vi "setTiming.vi"(8 "error in (no error)":errorcluster, 11 "niDAQmxDO in":refnum<class "niDAQmxDO.lvclass">) -> (0 "error out":errorcluster, 3 "niDAQmxDO out":refnum<class "niDAQmxDO.lvclass">)   [LabVIEW 2009, in "Hardware.lvlib" / "Channels.lvlib" / "niDAQmxDO.lvclass"]
doc: "need to add routings."
uses:
  niDAQmxDO.lvclass
  <vilib>/DAQmx/configure/timing.llb/DAQmx Timing (Sample Clock).vi
  C:/Program Files/National Instruments/LabVIEW 2009/resource/objmgr/daqmx.rc
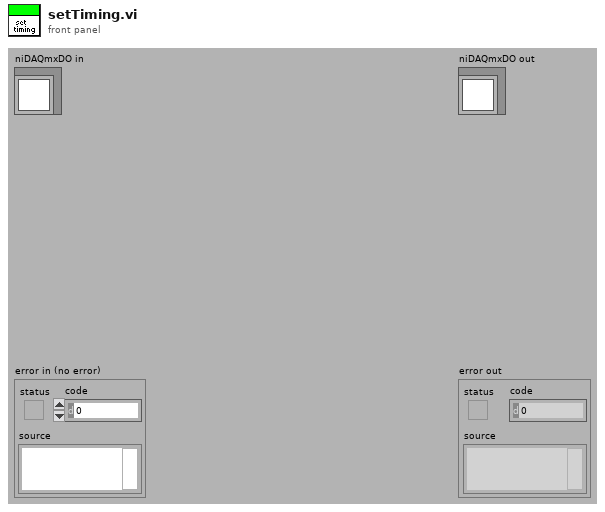
[diagram p1: front panel]
types:
  T1 = cluster{"Master Clock source":string, "Master Clock rate":dbl, "Start trigger line":string, "Scan rate":dbl, "Stop trigger line":string, "Sample Number":dbl}
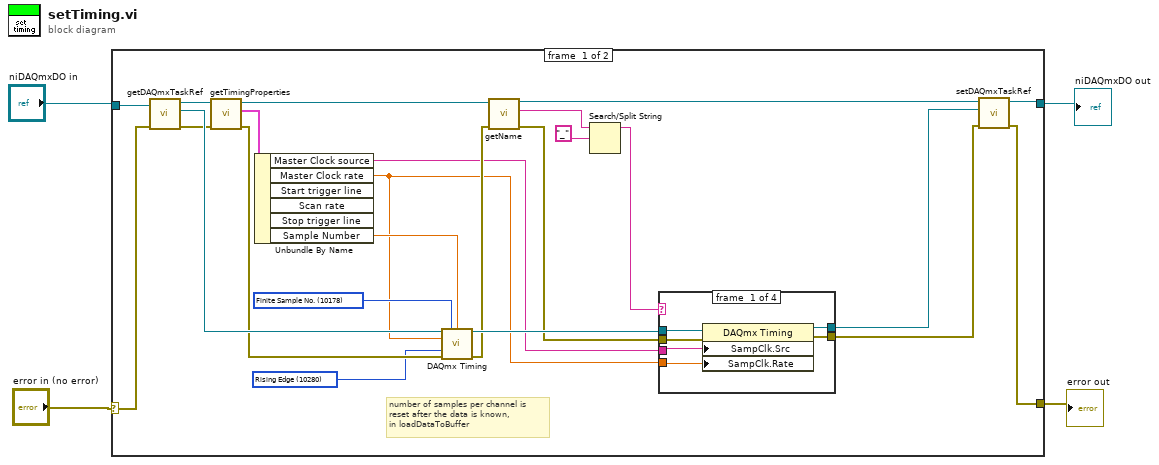
[diagram p0: block diagram]
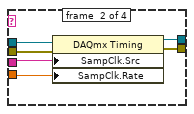
[diagram p2: hidden frame]
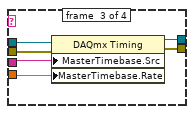
[diagram p3: hidden frame]
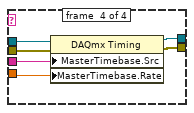
[diagram p4: hidden frame]
diagram:
  n1 = case shown="No Error" "error in (no error)" {
    selector: "error in (no error)" -> [w27 w54]
    tunnel: "niDAQmxDO in" -> [w28 w53]
    tunnel: [w20 w54] -> w2
    tunnel: [w19 w53] -> w1
    frame #0 {
      w16 = u16 10280 items=["Rising Edge"=10280]
      w22 = u16 10178 items=["Finite Sample No."=10178]
      # "number of samples per channel is\nreset after the data is known,\nin loadDataToBuffer"
      n2 = call "getDAQmxTaskRef.vi"("error in (no error)"=w27, "niDAQmxDO.lvclass in"=w28) -> ("error out"=w24:errorcluster, "DAQmx Task Ref"=w26:refnum<k21>, "niDAQmxDO.lvclass out"=w25:refnum<class "niDAQmxDO.lvclass">)  [unwired: 7 in]
      n3 = call-dynamic "getTimingProperties.vi"("error in (no error)"=w24, "DigitalOutput.lvclass in"=w25) -> ("error out"=w21:errorcluster, "Timing"=w23:T1, "DigitalOutput.lvclass out"=w15:refnum<class "niDAQmxDO.lvclass">)  [unwired: 7 in]
      n4 = Unbundle By Name(w23) -> ("Master Clock source"=w7:string, "Master Clock rate"=w11:dbl, "Sample Number"=w18:dbl)  [unwired: 3 out]
      n5 = call-poly <vilib>:"DAQmx Timing.vi"("task/channels in"=w26, "sample mode"=w22, "samples per channel"=w18, "rate"=w11, "active edge"=w16, "error in"=w21) -> ("task out"=w17:refnum<k21>, "error out"=w14:errorcluster)  [unwired: 8 in]
      n6 = call-dynamic "getName.vi"("error in (no error)"=w14, "DigitalOutput.lvclass in"=w15) -> ("error out"=w13:errorcluster, "name"=w9:string, "DigitalOutput.lvclass out"=w12:refnum<class "niDAQmxDO.lvclass">)  [unwired: 7 in]
      n7 = Search/Split String(string=w9, search string/char (-)="_") -> (substring before match=w8:string)  [unwired: 1 in, 2 out]
      n8 = case shown="\"UsbDAQ\"" w8 {
        tunnel: [w34 w40 w46 w52] -> w5
        tunnel: [w33 w39 w45 w51] -> w6
        tunnel: w11 -> [w32 w38 w44 w50]
        tunnel: w7 -> [w31 w37 w43 w49]
        tunnel: w17 -> [w30 w36 w42 w48]
        tunnel: w13 -> [w29 w35 w41 w47]
        frame #0 {
          n9 = property class="DAQmx Timing"(reference=w30, error in=w29, "SampClk.Src"=w31, "SampClk.Rate"=w32) -> (reference out=w34:refnum<k21>, error out=w33:errorcluster)
        }
        frame #1 {
          n10 = property class="DAQmx Timing"(reference=w36, error in=w35, "SampClk.Src"=w37, "SampClk.Rate"=w38) -> (reference out=w40:refnum<k21>, error out=w39:errorcluster)
        }
        frame #2 {
          n11 = property class="DAQmx Timing"(reference=w42, error in=w41, "MasterTimebase.Src"=w43, "MasterTimebase.Rate"=w44) -> (reference out=w46:refnum<k21>, error out=w45:errorcluster)
        }
        frame #3 {
          n12 = property class="DAQmx Timing"(reference=w48, error in=w47, "MasterTimebase.Src"=w49, "MasterTimebase.Rate"=w50) -> (reference out=w52:refnum<k21>, error out=w51:errorcluster)
        }
      }
      n13 = call "setDAQmxTaskRef.vi"("error in (no error)"=w6, "DAQmx Task Ref"=w5, "niDAQmxDO.lvclass in"=w12) -> ("error out"=w20:errorcluster, "niDAQmxDO.lvclass out"=w19:refnum<class "niDAQmxDO.lvclass">)  [unwired: 7 in]
    }
    frame #1 {
    }
  }
  "error out" <- w2
  "niDAQmxDO out" <- w1
